vi "I2C Close Channel.vi"(8 "error in (no error)":errorcluster, 11 "handle":u64) -> (0 "error out":errorcluster, 2 "function return":u32, 3 "handle out":u32)   [LabVIEW 2024, in "libMPSSE-I2C.lvlib"]
doc: "FTDI_API FT_STATUS SPI_CloseChannel(FT_HANDLE handle);"
uses:
  libMPSSE-I2C.lvlib
  libmpsse.dll
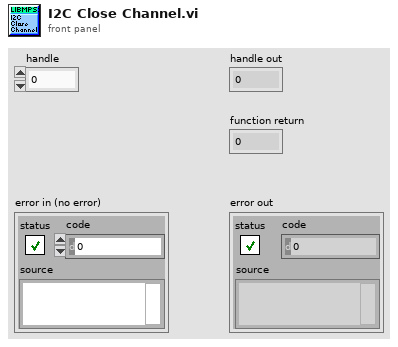
[diagram p1: front panel]
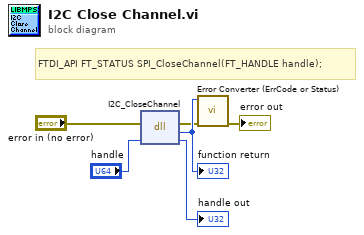
[diagram p0: block diagram]
diagram:
  # "FTDI_API FT_STATUS SPI_CloseChannel(FT_HANDLE handle);"
  n1 = dll-call lib="C:/Sandbox/sm_6576_001_RIB_Sequencer/I2C/libmpsse.dll" fn="I2C_CloseChannel"(error in="error in (no error)", "handle"="handle") -> (error out=w3:errorcluster, "return type"=w6:u64, "handle"=→"handle out":u64)  [unwired: 2 in, 1 out]
  "function return" <- w6
  n2 = call "Error Converter (ErrCode or Status).vi"("error in (no error)"=w3, "error code"=w6) -> ("error out"=→"error out":errorcluster)  [unwired: 9 in]
